vi "initialize - lan.vi"(8 "error in (no error)":errorcluster, 10 "controller number(0)":u32, 11 "ip":string) -> (0 "error out":errorcluster)   [LabVIEW 2024, in "atsj peakcan basic.lvlib"]
doc: "Initializes a PCAN LAN bus (channel) with bitrate adaptation enabled (automatic bitrate selection). This VI supports initialization of both Classical CAN and CAN FD devices.\n\nCopyright (c) 2025 ATSJ (www.atsj.eu)"
uses:
  atsj peakcan basic.lvlib
  device type.ctl
  bitrate.ctl
  fd bitrate.ctl
  clock frequency.ctl
  fd bitrate parameters.ctl
  get channel handle - by device controller index.vi
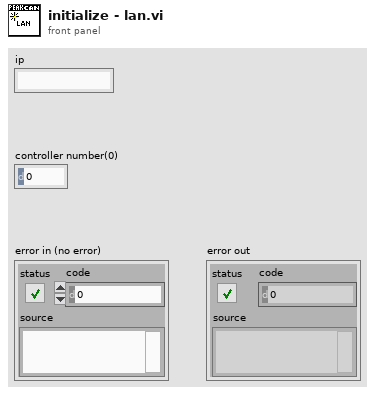
[diagram p1: front panel]
types:
  T1 = typedef "atsj peakcan basic.lvlib/device type.ctl" = enum8{"ISA", "DNG", "PCI", "USB", "PCC", "LAN"}
  T2 = typedef "atsj peakcan basic.lvlib/bitrate.ctl" = enum16{"RATE_1Mbps", "RATE_800kbps", "RATE_500kbps", "RATE_250kbps", "RATE_125kbps", "RATE_100kbps", "RATE_95kbps", "RATE_83kbps", "RATE_50kbps", "RATE_47kbps", "RATE_33kbps", "RATE_20kbps", "RATE_10kbps", "RATE_5kbps"}
  T3 = typedef "atsj peakcan basic.lvlib/fd bitrate.ctl" = cluster{"clock frequency":T4, "nominal bitrate":T5, "data bitrate":T5}
  T4 = typedef "atsj peakcan basic.lvlib/clock frequency.ctl" = enum16{"CLOCK_80MHz", "CLOCK_60MHz", "CLOCK_40MHz", "CLOCK_30MHz", "CLOCK_24MHz", "CLOCK_20MHz"}
  T5 = typedef "atsj peakcan basic.lvlib/fd bitrate parameters.ctl" = cluster{"bitrate prescaler":u16, "time segment 1":u16, "time segment 2":u16, "sync jump width":u16}
  T6 = typedef "atsj peakcan basic.lvlib/features.ctl" = cluster{"fd capable":bool, "delay capable":bool, "io capable":bool}
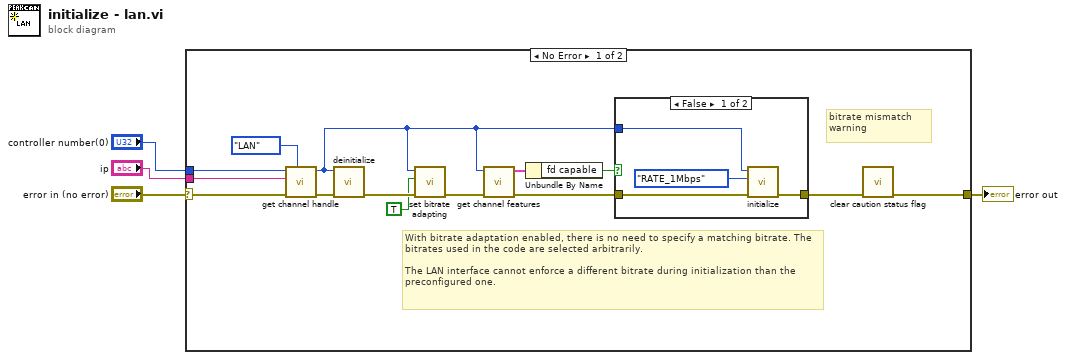
[diagram p0: block diagram]
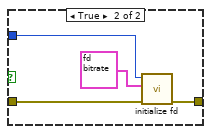
[diagram p2: hidden frame]
diagram:
  n1 = case shown="No Error" "error in (no error)" {
    selector: "error in (no error)" -> [w6 w27]
    tunnel: "ip" -> [w9 _]
    tunnel: "controller number(0)" -> [w8 _]
    tunnel: [w5 w27] -> w1
    frame No Error {
      # "bitrate mismatch warning"
      # "With bitrate adaptation enabled, there is no need to specify a matching bitrate. The bitrates used in the code are selected arbitrarily.\n\nThe LAN interface cannot enforce a different bitrate during initialization than the preconfigured one."
      n2 = call-poly "get channel handle.vi"("device type"=device_type."LAN", "error in (no error)"=w6, "ip (\"\")"=w9, "controller number(0)"=w8) -> ("error out"=w11:errorcluster, "channel handle"=w7:u16)  [unwired: 6 in]
      n3 = call "deinitialize.vi"("error in (no error)"=w11, "channel handle (0:all)"=w7) -> ("error out"=w18:errorcluster)  [unwired: 9 in]
      n4 = call "set bitrate adapting.vi"("error in (no error)"=w18, "enable (F)"=TRUE, "channel handle"=w7) -> ("error out"=w14:errorcluster)  [unwired: 8 in]
      n5 = call "get channel features.vi"("error in (no error)"=w14, "channel handle"=w7) -> ("error out"=w16:errorcluster, "features"=w17:T6)  [unwired: 8 in]
      n6 = Unbundle By Name(w17) -> ("fd capable"=w15:bool)
      n7 = case shown="False" w15 {
        tunnel: w16 -> [w22 w26]
        tunnel: w7 -> [w21 w25]
        tunnel: [w20 w24] -> w12
        frame False {
          n8 = call "initialize.vi"("error in (no error)"=w22, "bitrate"=bitrate."RATE_1Mbps", "channel handle"=w21) -> ("error out"=w20:errorcluster)  [unwired: 8 in]
        }
        frame True {
          n9 = call "initialize fd.vi"("error in (no error)"=w26, "bitrate"=T3 {"clock frequency"=enum."CLOCK_80MHz", "nominal bitrate"={"bitrate prescaler"=2, "time segment 1"=63, "time segment 2"=16, "sync jump width"=16}, "data bitrate"={"bitrate prescaler"=2, "time segment 1"=15, "time segment 2"=4, "sync jump width"=4}}, "channel handle"=w25) -> ("error out"=w24:errorcluster)  [unwired: 8 in]
        }
      }
      n10 = call "clear caution status flag.vi"("error in (no error)"=w12) -> ("error out"=w5:errorcluster)  [unwired: 10 in]
    }
    frame Error {
    }
  }
  "error out" <- w1
